vi "LWXPS_ZygoSetPEGParams.vi"(0 "End PEG region":i64, 1 "Start PEG region":i64, 2 "XPS Reference IN":refnum<k24>, 5 "Increment value 1":u32, 7 "Number of PEG events 1":i64, 9 "Increment value 2":u32, 11 "Number of PEG events 2":i64, 12 "PEG control":i32, 13 "LabVIEW error IN":errorcluster) -> (4 "XPS Reference OUT":refnum<k24>, 6 "Returned error code":i32, 8 "XPS Error String":string, 15 "LabVIEW error OUT":errorcluster)   [LabVIEW 2014]
uses:
  D:/XPSQ8_LabView_Library/Development/Source/Dll/Newport.XPS.CommandInterface.dll
  Dll/Newport.XPS.CommandInterface.dll
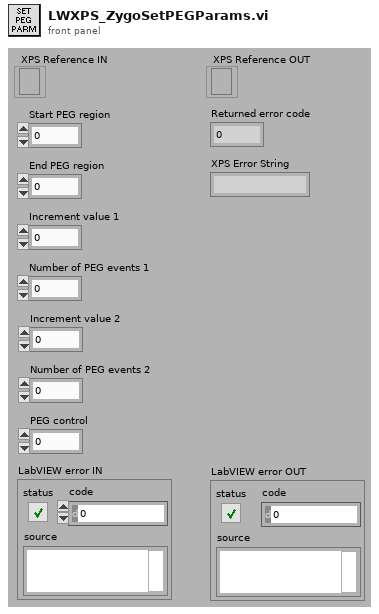
[diagram p1: front panel]
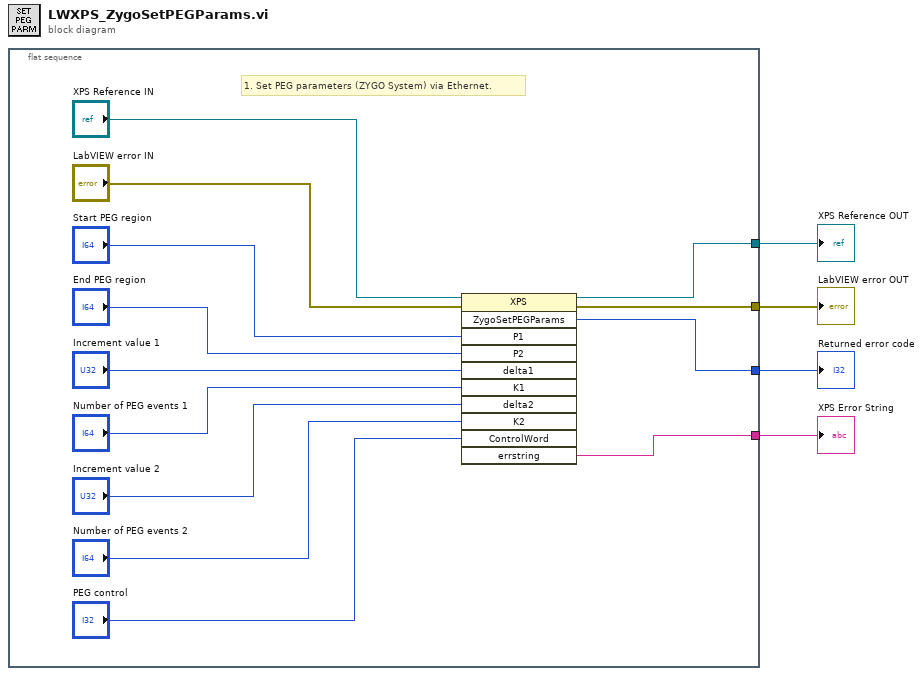
[diagram p0: block diagram]
diagram:
  n1 = flat-sequence {
    tunnel: [w15] -> w4
    tunnel: [w14] -> w3
    tunnel: [w16] -> w2
    tunnel: [w11] -> w1
    frame #0 {
      # "1. Set PEG parameters (ZYGO System) via Ethernet."
      n2 = invoke class="XPS" method="ZygoSetPEGParams"(reference="XPS Reference IN", error in="LabVIEW error IN", "P1"="Start PEG region", "P2"="End PEG region", "delta1"="Increment value 1", "K1"="Number of PEG events 1", "delta2"="Increment value 2", "K2"="Number of PEG events 2", "ControlWord"="PEG control") -> (reference out=w15:refnum<k24>, error out=w14:errorcluster, "ZygoSetPEGParams"=w16:i32, "errstring"=w11:string)  [unwired: 2 in, 7 out]
    }
  }
  "XPS Error String" <- w1
  "XPS Reference OUT" <- w4
  "LabVIEW error OUT" <- w3
  "Returned error code" <- w2
